vi "CheckPacketChecksum.vi"(1 "Expected Packet Length":i32, 2 "Buffer":string) -> (0 "Packet Valid":bool)   [LabVIEW 2015, in "navX Library v3.lvlib" / "navX - SERIAL.lvclass"]
uses:
  navX - SERIAL.lvclass
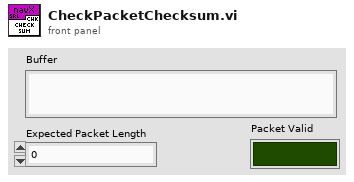
[diagram p1: front panel]
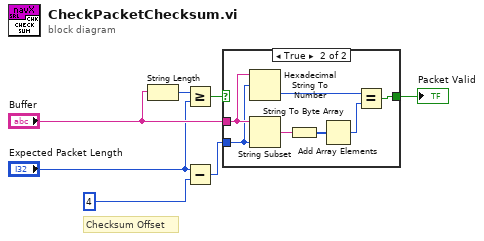
[diagram p0: block diagram]
diagram:
  # "Checksum Offset"
  n1 = String Length(string="Buffer") -> (length=w3:i32)
  n2 = Greater Or Equal?(x=w3, y="Expected Packet Length") -> (x >= y?=w1:bool)
  n3 = Subtract(x="Expected Packet Length", y=4) -> (x-y=w6:i32)
  n4 = case shown="True" w1 {
    selector: w1 -> [w8 _]
    tunnel: w6 -> [_ w12]
    tunnel: [w8 w9] -> w4
    tunnel: "Buffer" -> [_ w13]
    frame False {
    }
    frame True {
      n5 = Hexadecimal String To Number(string=w13, offset=w12) -> (number=w10:u32)  [unwired: 1 in, 1 out]
      n6 = String Subset(string=w13, length (rest)=w12) -> (substring=w15:string)  [unwired: 1 in]
      n7 = String To Byte Array(string=w15) -> (unsigned byte array=w14:u8[])
      n8 = Add Array Elements(numeric array=w14) -> (sum=w11:u8)
      n9 = Equal?(x=w10, y=w11) -> (x = y?=w9:bool)
    }
  }
  "Packet Valid" <- w4
